vi "SP Calculate TYX.vi"(10 "SP Array (SXX, SXY, SYX, SYY)":cdb[](array[numeric])) -> (2 "TYX":cdb)   [LabVIEW 2011]
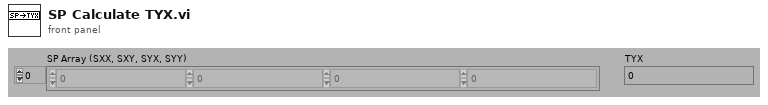
[diagram p1: front panel]
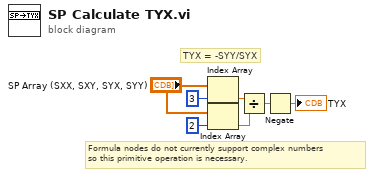
[diagram p0: block diagram]
diagram:
  # "TYX = -SYY/SYX"
  # "Formula nodes do not currently support complex numbers\nso this primitive operation is necessary."
  n1 = Index Array(array="SP Array (SXX, SXY, SYX, SYY)", index=3) -> (element=w2:cdb)
  n2 = Index Array(array="SP Array (SXX, SXY, SYX, SYY)", index=2) -> (element=w1:cdb)
  n3 = Divide(x=w2, y=w1) -> (x/y=w4:cdb)
  n4 = Negate(x=w4) -> (-x=→"TYX":cdb)
